vi "Array_Builder_Dual.vi"(4 "OSC Number":i16, 6 "Cycle Length":dbl, 8 "Array In 2":dbl[](array[numeric]), 9 "Input 2":dbl, 10 "Array In":dbl[](array[numeric]), 11 "Input":dbl) -> (0 "Array Out Main 2":dbl[](array[numeric]), 2 "Array Out Main":dbl[](array[numeric]))   [LabVIEW 2014]
panel:
  # "Moving Average VI"
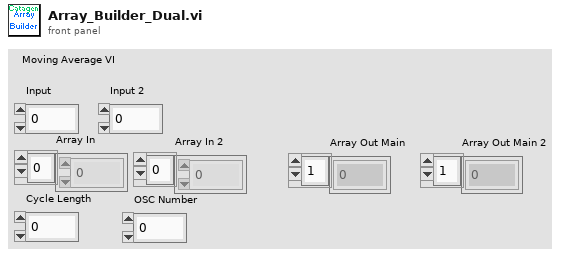
[diagram p1: front panel]
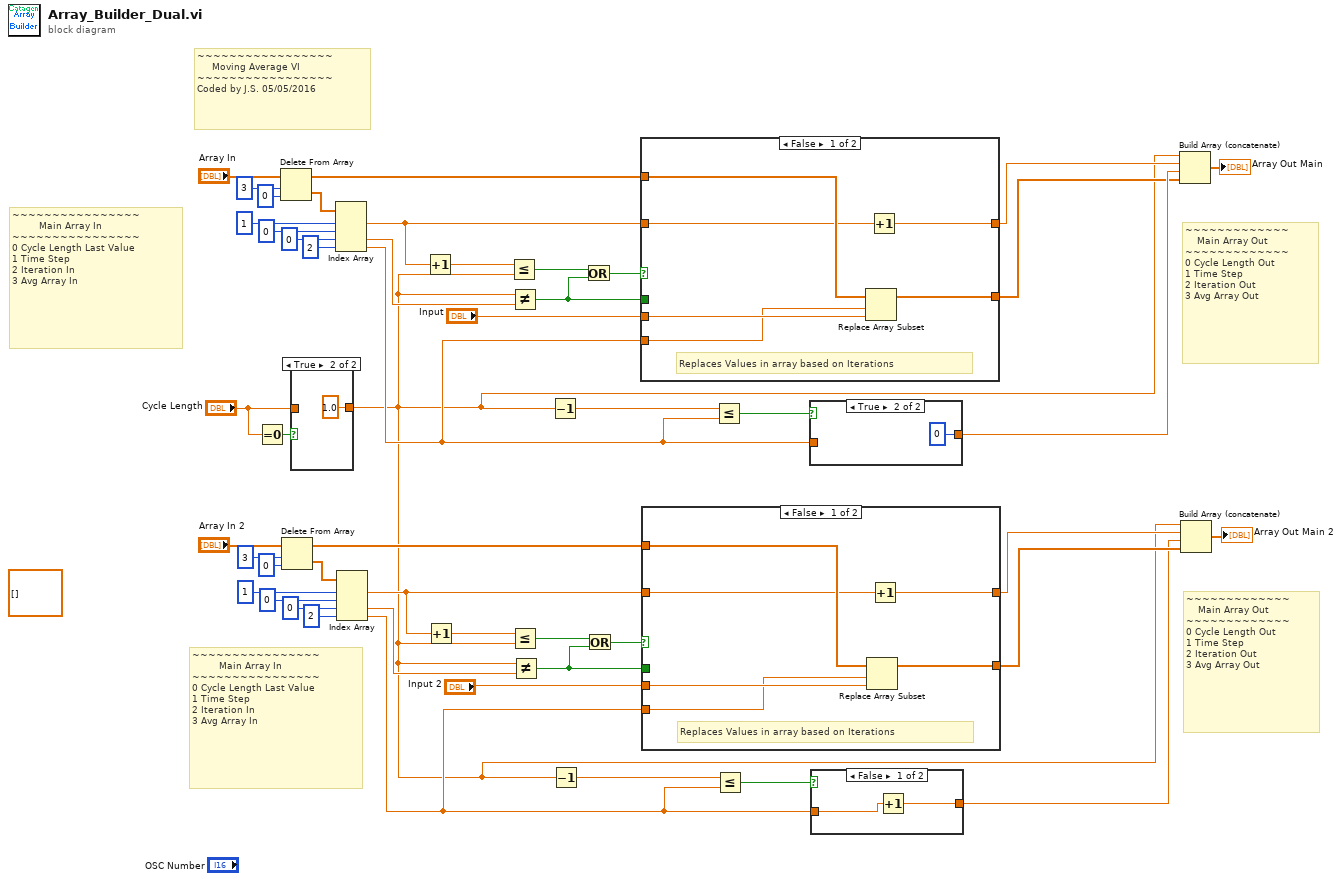
[diagram p0: block diagram]
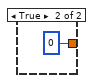
[diagram p3: hidden frame]
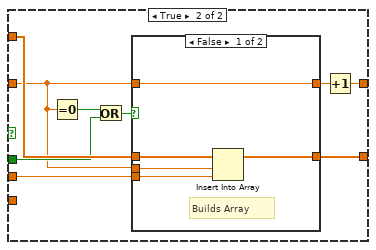
[diagram p4: hidden frame]
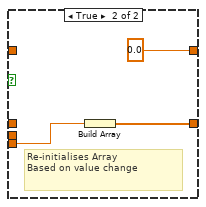
[diagram p5: hidden frame]
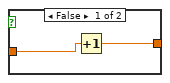
[diagram p6: hidden frame]
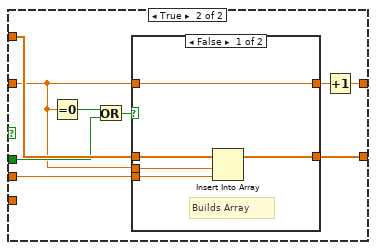
[diagram p7: hidden frame]
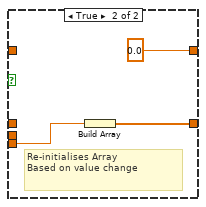
[diagram p8: hidden frame]
diagram:
  (unwired) dbl[][] [] ("2D array")
  # "~~~~~~~~~~~~~~~~\n         Main Array In\n~~~~~~~~~~~~~~~~\n0 Cycle Length Last Value\n1 Time Step\n2 Iteration In\n3 Avg Array In"
  # "~~~~~~~~~~~~~\n    Main Array Out\n~~~~~~~~~~~~~\n0 Cycle Length Out\n1 Time Step\n2 Iteration Out\n3 Avg Array Out"
  # "~~~~~~~~~~~~~~~~\n         Main Array In\n~~~~~~~~~~~~~~~~\n0 Cycle Length Last Value\n1 Time Step\n2 Iteration In\n3 Avg Array In"
  # "~~~~~~~~~~~~~\n    Main Array Out\n~~~~~~~~~~~~~\n0 Cycle Length Out\n1 Time Step\n2 Iteration Out\n3 Avg Array Out"
  # "~~~~~~~~~~~~~~~~~\n     Moving Average VI \n~~~~~~~~~~~~~~~~~\nCoded by J.S. 05/05/2016"
  n1 = Equal To 0?(x="Cycle Length") -> (x = 0?=w3:bool)
  n2 = Delete From Array(array="Array In", length=3, index=0) -> (deleted portion=w40:dbl[], array with subset deleted=w36:dbl[])
  n3 = Delete From Array(array="Array In 2", length=3, index=0) -> (deleted portion=w14:dbl[], array with subset deleted=w17:dbl[])
  n4 = case shown="True" w3 {
    tunnel: "Cycle Length" -> [w50 _]
    tunnel: [w50 1.0 ("Cycle Length")] -> w1
    frame False {
    }
    frame True {
    }
  }
  n5 = Index Array(array=w40, index #1=1 ("index"), index #2=0 ("index"), index #3=0 ("index"), index #4=2 ("index")) -> (element #1=w29:dbl, element #3=w33:dbl, element #4=w31:dbl)  [unwired: 1 out]
  n6 = Index Array(array=w14, index #1=1 ("index"), index #2=0 ("index"), index #3=0 ("index"), index #4=2 ("index")) -> (element #1=w24:dbl, element #3=w20:dbl, element #4=w22:dbl)  [unwired: 1 out]
  n7 = Increment(x=w29) -> (x+1=w28:dbl)
  n8 = Increment(x=w24) -> (x+1=w25:dbl)
  n9 = Less Or Equal?(x=w28, y=w1) -> (x <= y?=w48:bool)
  n10 = Not Equal?(x=w1, y=w33) -> (x != y?=w46:bool)
  n11 = Less Or Equal?(x=w25, y=w1) -> (x <= y?=w8:bool)
  n12 = Not Equal?(x=w1, y=w20) -> (x != y?=w9:bool)
  n13 = Decrement(x=w1) -> (x-1=w44:dbl)
  n14 = Decrement(x=w1) -> (x-1=w11:dbl)
  n15 = Or(x=w48, y=w46) -> (x .or. y?=w49:bool)
  n16 = Or(x=w8, y=w9) -> (x .or. y?=w7:bool)
  n17 = case shown="False" w49 {
    tunnel: "Input" -> [w55 w65]
    tunnel: [w56 w64] -> w42
    tunnel: w36 -> [w57 w66]
    tunnel: w31 -> [w54 _]
    tunnel: w29 -> [w53 w60]
    tunnel: w46 -> [_ w63]
    tunnel: [w52 w59] -> w27
    frame False {
      # "Replaces Values in array based on Iterations"
      n18 = Replace Array Subset(array=w57, new element=w55, index=w54) -> (w56:dbl[])
      n19 = Increment(x=w53) -> (x+1=w52:dbl)
    }
    frame True {
      n20 = Equal To 0?(x=w60) -> (x = 0?=w61:bool)
      n21 = Or(x=w61, y=w63) -> (x .or. y?=w62:bool)
      n22 = case shown="False" w62 {
        tunnel: w66 -> [w71 _]
        tunnel: w65 -> [w70 w73]
        tunnel: [w69 w74] -> w64
        tunnel: w60 -> [w68 _]
        tunnel: w60 -> [w67 _]
        tunnel: [w67 0.0] -> w58
        frame False {
          # "Builds Array"
          n23 = Insert Into Array(array=w71, index=w68, new element=w70) -> (w69:dbl[])
        }
        frame True {
          # "Re-initialises Array\nBased on value change"
          n24 = Build Array(w73) -> (w74:dbl[])
        }
      }
      n25 = Increment(x=w58) -> (x+1=w59:dbl)
    }
  }
  n26 = case shown="False" w7 {
    tunnel: "Input 2" -> [w78 w88]
    tunnel: [w79 w87] -> w13
    tunnel: w17 -> [w80 w89]
    tunnel: w22 -> [w77 _]
    tunnel: w24 -> [w76 w83]
    tunnel: w9 -> [_ w86]
    tunnel: [w75 w82] -> w26
    frame False {
      # "Replaces Values in array based on Iterations"
      n27 = Replace Array Subset(array=w80, new element=w78, index=w77) -> (w79:dbl[])
      n28 = Increment(x=w76) -> (x+1=w75:dbl)
    }
    frame True {
      n29 = Equal To 0?(x=w83) -> (x = 0?=w84:bool)
      n30 = Or(x=w84, y=w86) -> (x .or. y?=w85:bool)
      n31 = case shown="False" w85 {
        tunnel: w89 -> [w94 _]
        tunnel: w88 -> [w93 w96]
        tunnel: [w92 w97] -> w87
        tunnel: w83 -> [w91 _]
        tunnel: w83 -> [w90 _]
        tunnel: [w90 0.0] -> w81
        frame False {
          # "Builds Array"
          n32 = Insert Into Array(array=w94, index=w91, new element=w93) -> (w92:dbl[])
        }
        frame True {
          # "Re-initialises Array\nBased on value change"
          n33 = Build Array(w96) -> (w97:dbl[])
        }
      }
      n34 = Increment(x=w81) -> (x+1=w82:dbl)
    }
  }
  n35 = Less Or Equal?(x=w44, y=w31) -> (x <= y?=w45:bool)
  n36 = Less Or Equal?(x=w11, y=w22) -> (x <= y?=w10:bool)
  n37 = case shown="True" w45 {
    tunnel: [w99 i64 0] -> w43
    tunnel: w31 -> [w98 _]
    frame False {
      n38 = Increment(x=w98) -> (x+1=w99:dbl)
    }
    frame True {
    }
  }
  n39 = case shown="False" w10 {
    tunnel: [w102 i64 0] -> w12
    tunnel: w22 -> [w101 _]
    frame False {
      n40 = Increment(x=w101) -> (x+1=w102:dbl)
    }
    frame True {
    }
  }
  n41 = Build Array (concatenate)(w1, w27, w43, w42) -> (→"Array Out Main":dbl[])
  n42 = Build Array (concatenate)(w1, w26, w12, w13) -> (→"Array Out Main 2":dbl[])
